vi "SRV_VIG_Camera.vi"(0 "Camera":bool, 9 "Images Directory Path":path, 12 "Method (Get)":enum16{"Get", "Set"}(ring)) -> (4 "Camera?":bool, 10 "Images Directory Path out":path)   [LabVIEW 2014]
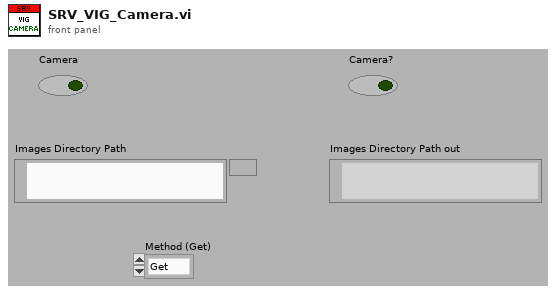
[diagram p1: front panel]
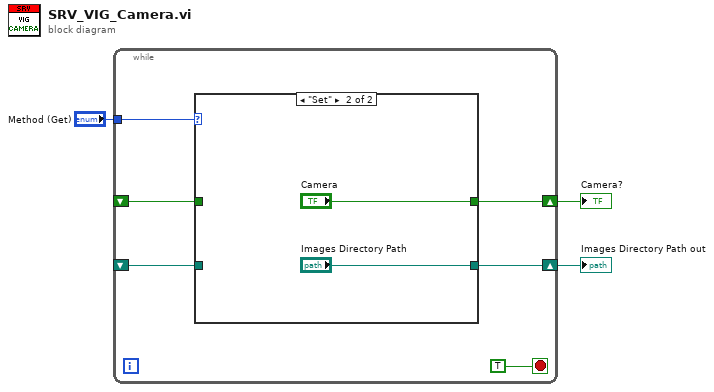
[diagram p0: block diagram]
diagram:
  n1 = while {
    tunnel: "Method (Get)" -> [w9]
    shift-right: [w7] -> w2
    shift-left: _ -> [w8]
    shift-right: [w5] -> w1
    shift-left: _ -> [w4]
    stop <- TRUE stop-if-true
    n2 = case shown="\"Set\"" w9 {
      tunnel: w8 -> [w11 _]
      tunnel: [w11 "Camera"] -> w7
      tunnel: [w10 "Images Directory Path"] -> w5
      tunnel: w4 -> [w10 _]
      frame "Get" {
      }
      frame "Set" {
      }
    }
  }
  "Camera?" <- w2
  "Images Directory Path out" <- w1
